vi "filterCalcTimerValues.vi"(11 "speed(steps/Sec)":u32=1000) -> (3 "data":u8[](array[numeric]), 5 "Timer":u16, 7 "MUL":u8)   [LabVIEW 2018]
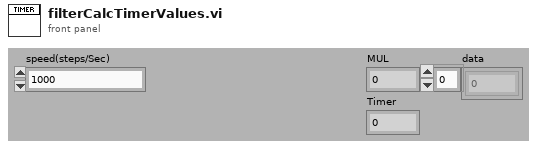
[diagram p1: front panel]
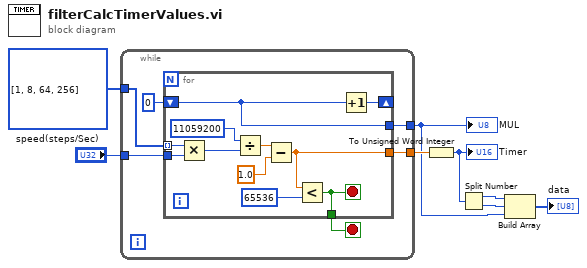
[diagram p0: block diagram]
diagram:
  n1 = while {
    tunnel: i32[] [1, 8, 64, 256] -> [w14]
    tunnel: "speed(steps/Sec)" -> [w13]
    tunnel: [w11] -> w6
    tunnel: [w10] -> w2
    stop <- w9 stop-if-true
    n2 = for {
      tunnel: w14 -> [w24] mode=indexing
      shift-right: [w25] -> _
      shift-left: u8 0 -> [w17]
      tunnel: w13 -> [w23]
      tunnel: [w17] -> w10
      tunnel: [w16] -> w11
      tunnel: [w15] -> w9
      stop <- w15 stop-if-true
      n3 = Multiply(x=w24, y=w23) -> (x*y=w22:u32)
      n4 = Divide(x=11059200, y=w22) -> (x/y=w20:dbl)
      n5 = Subtract(x=w20, y=1.0) -> (x-y=w16:dbl)
      n6 = Less?(x=w16, y=65536) -> (x < y?=w15:bool)
      n7 = Increment(x=w17) -> (x+1=w25:u8)
    }
  }
  "MUL" <- w2
  n8 = To Unsigned Word Integer(number=w6) -> (unsigned 16bit integer=w5:u16)
  "Timer" <- w5
  n9 = Split Number(x=w5) -> (hi(x)=w4:u8, lo(x)=w3:u8)
  n10 = Build Array(w4, w3, w2) -> (→"data":u8[])
